vi "subvi_Identification_tdms.vi"(8 "Error In":errorcluster caption="에러 입력", 11 "Path in":path) -> (0 "Error Out":errorcluster caption="에러 출력", 2 "TDMS_info":T1, 3 "Path out":path)   [LabVIEW 2016]
panel:
  in  "숫자형 컨트롤 2":i32
  in  "숫자형 컨트롤":u64
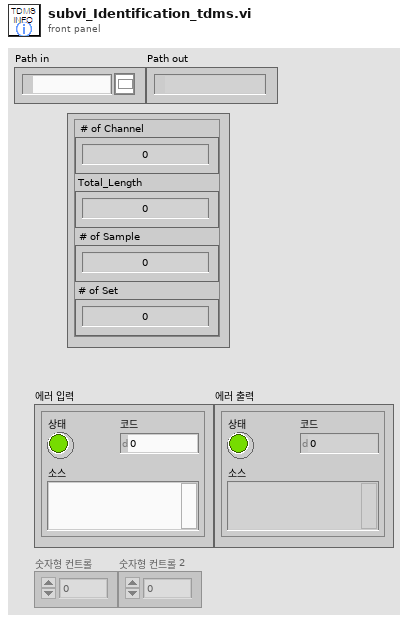
[diagram p1: front panel]
types:
  T1 = cluster{"# of Channel":i32, "Total_Length":u64, "# of Sample":i32, "# of Set":i32}
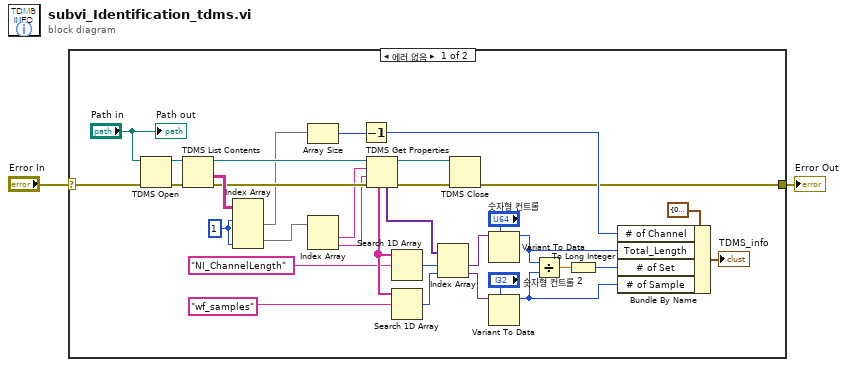
[diagram p0: block diagram]
diagram:
  n1 = case shown="에러 없음" "Error In" {
    selector: "Error In" -> [w6 w36]
    tunnel: [w5 w36] -> w1
    frame No Error {
      w15 = 1 ("인덱스 (행)")
      n2 = TDMS Open(8:w6, 11:"Path in") -> (0:w30:errorcluster, 3:w33:refnum<k34>)  [unwired: 5 in]
      n3 = TDMS List Contents(4:w30, 7:w33) -> (0:w29:errorcluster, 1:w32:string[][], 3:w31:refnum<k34>)  [unwired: 1 in, 1 out]
      n4 = Index Array(array=w32, index (row) #1=w15, index (col) #2=w15) -> (element #1=w13:string[], element #2=w14:string[])  [unwired: 2 in]
      n5 = Array Size(array=w13) -> (size(s)=w16:i32)
      n6 = Index Array(array=w14) -> (element #1=w28:string, element #2=w27:string)  [unwired: 2 in]
      n7 = Decrement(x=w16) -> (x-1=w8:i32)
      n8 = TDMS Get Properties(8:w29, 9:w27, 10:w28, 11:w31) -> (0:w34:errorcluster, 3:w35:refnum<k34>, 4:w17:variant[], 6:w26:string[])  [unwired: 2 in, 2 out]
      n9 = Search 1D Array(1D array=w26, element="NI_ChannelLength") -> (index of element=w23:i32)  [unwired: 1 in]
      n10 = Search 1D Array(1D array=w26, element="wf_samples") -> (index of element=w22:i32)  [unwired: 1 in]
      n11 = Index Array(array=w17, index #1=w23, index #2=w22) -> (element #1=w21:variant, element #2=w18:variant)
      n12 = TDMS Close(8:w34, 11:w35) -> (0:w5:errorcluster)  [unwired: 1 out]
      n13 = Variant To Data(type="숫자형 컨트롤", Variant=w21) -> (data=w9:u64)  [unwired: 1 in, 1 out]
      n14 = Variant To Data(type="숫자형 컨트롤 2", Variant=w18) -> (data=w11:i32)  [unwired: 1 in, 1 out]
      n15 = Divide(x=w9, y=w11) -> (x/y=w10:dbl)
      n16 = To Long Integer(number=w10) -> (32bit integer=w3:i32)
      n17 = Bundle By Name(cluster=T1 {"# of Channel"=0, "Total_Length"=0, "# of Sample"=0, "# of Set"=0} ("TDMS_info 2"), "# of Channel"=w8, "Total_Length"=w9, "# of Set"=w3, "# of Sample"=w11) -> (→"TDMS_info":T1)
      "Path out" <- "Path in"
    }
    frame Error {
    }
  }
  "Error Out" <- w1
